vi "Convert Subset to String.vi"(7 "Image Units":T1, 8 "Bottom":i16, 9 "Right":i16, 10 "Top":i16, 11 "Left":i16) -> (3 "Subset String":string)   [LabVIEW 2020, in "MacroAssert.lvlib" / "Image Assertion.lvclass"]
uses:
  Image Assertion.lvclass
  Image Assertion.lvclass/Image Assertion.ctl
  Image Units.ctl
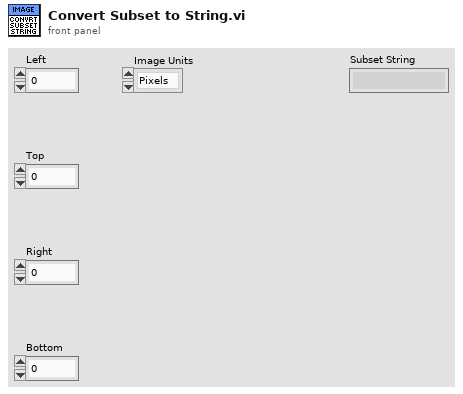
[diagram p1: front panel]
types:
  T1 = typedef "MacroAssert.lvlib/Image Assertion.lvclass/Image Units.ctl" = enum16{"Pixels", "Percent"}
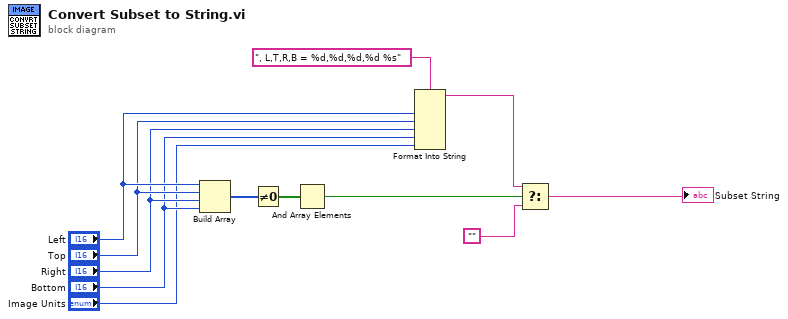
[diagram p0: block diagram]
diagram:
  n1 = Build Array("Left", "Top", "Right", "Bottom") -> (w12:i16[])
  n2 = Not Equal To 0?(x=w12) -> (x != 0?=w11:bool[])
  n3 = And Array Elements(Boolean array=w11) -> (logical AND=w4:bool)
  n4 = Format Into String(format string=", L,T,R,B = %d,%d,%d,%d %s", "Left", "Top", "Right", "Bottom", "Image Units") -> (resulting string=w3:string)  [unwired: 2 in, 1 out]
  n5 = Select(t=w3, s=w4, f="") -> (s? t:f=→"Subset String":string)
